vi "Serial.Get Com Port Device List.vi"(8 "error in":errorcluster) -> (0 "error out":errorcluster, 3 "Ports":T1(array[cluster]))   [LabVIEW 2018]
uses:
  <vilib>/KATE/Time/Time Utils.lvlib
panel:
  out "Duration(s)":dbl
  out "STD Error":string
  out "STD Out":string
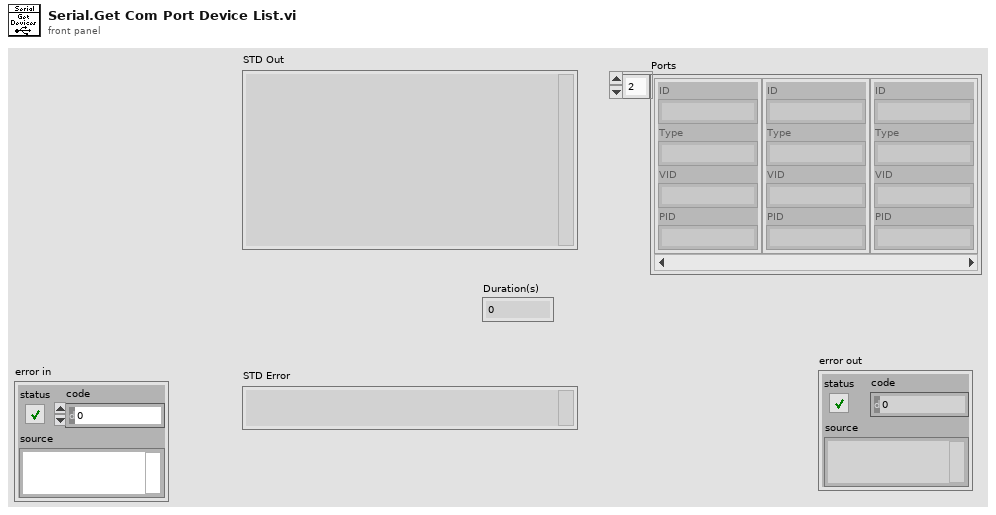
[diagram p1: front panel]
types:
  T1 = cluster{"ID":string, "Type":string, "VID":string, "PID":string}[]
  T2 = cluster{"ID":string, "Type":string, "VID":string, "PID":string}
  T3 = cluster{"STDIO":string, "Ports":cluster{"ID":string, "Type":string, "VID":string, "PID":string}[]}
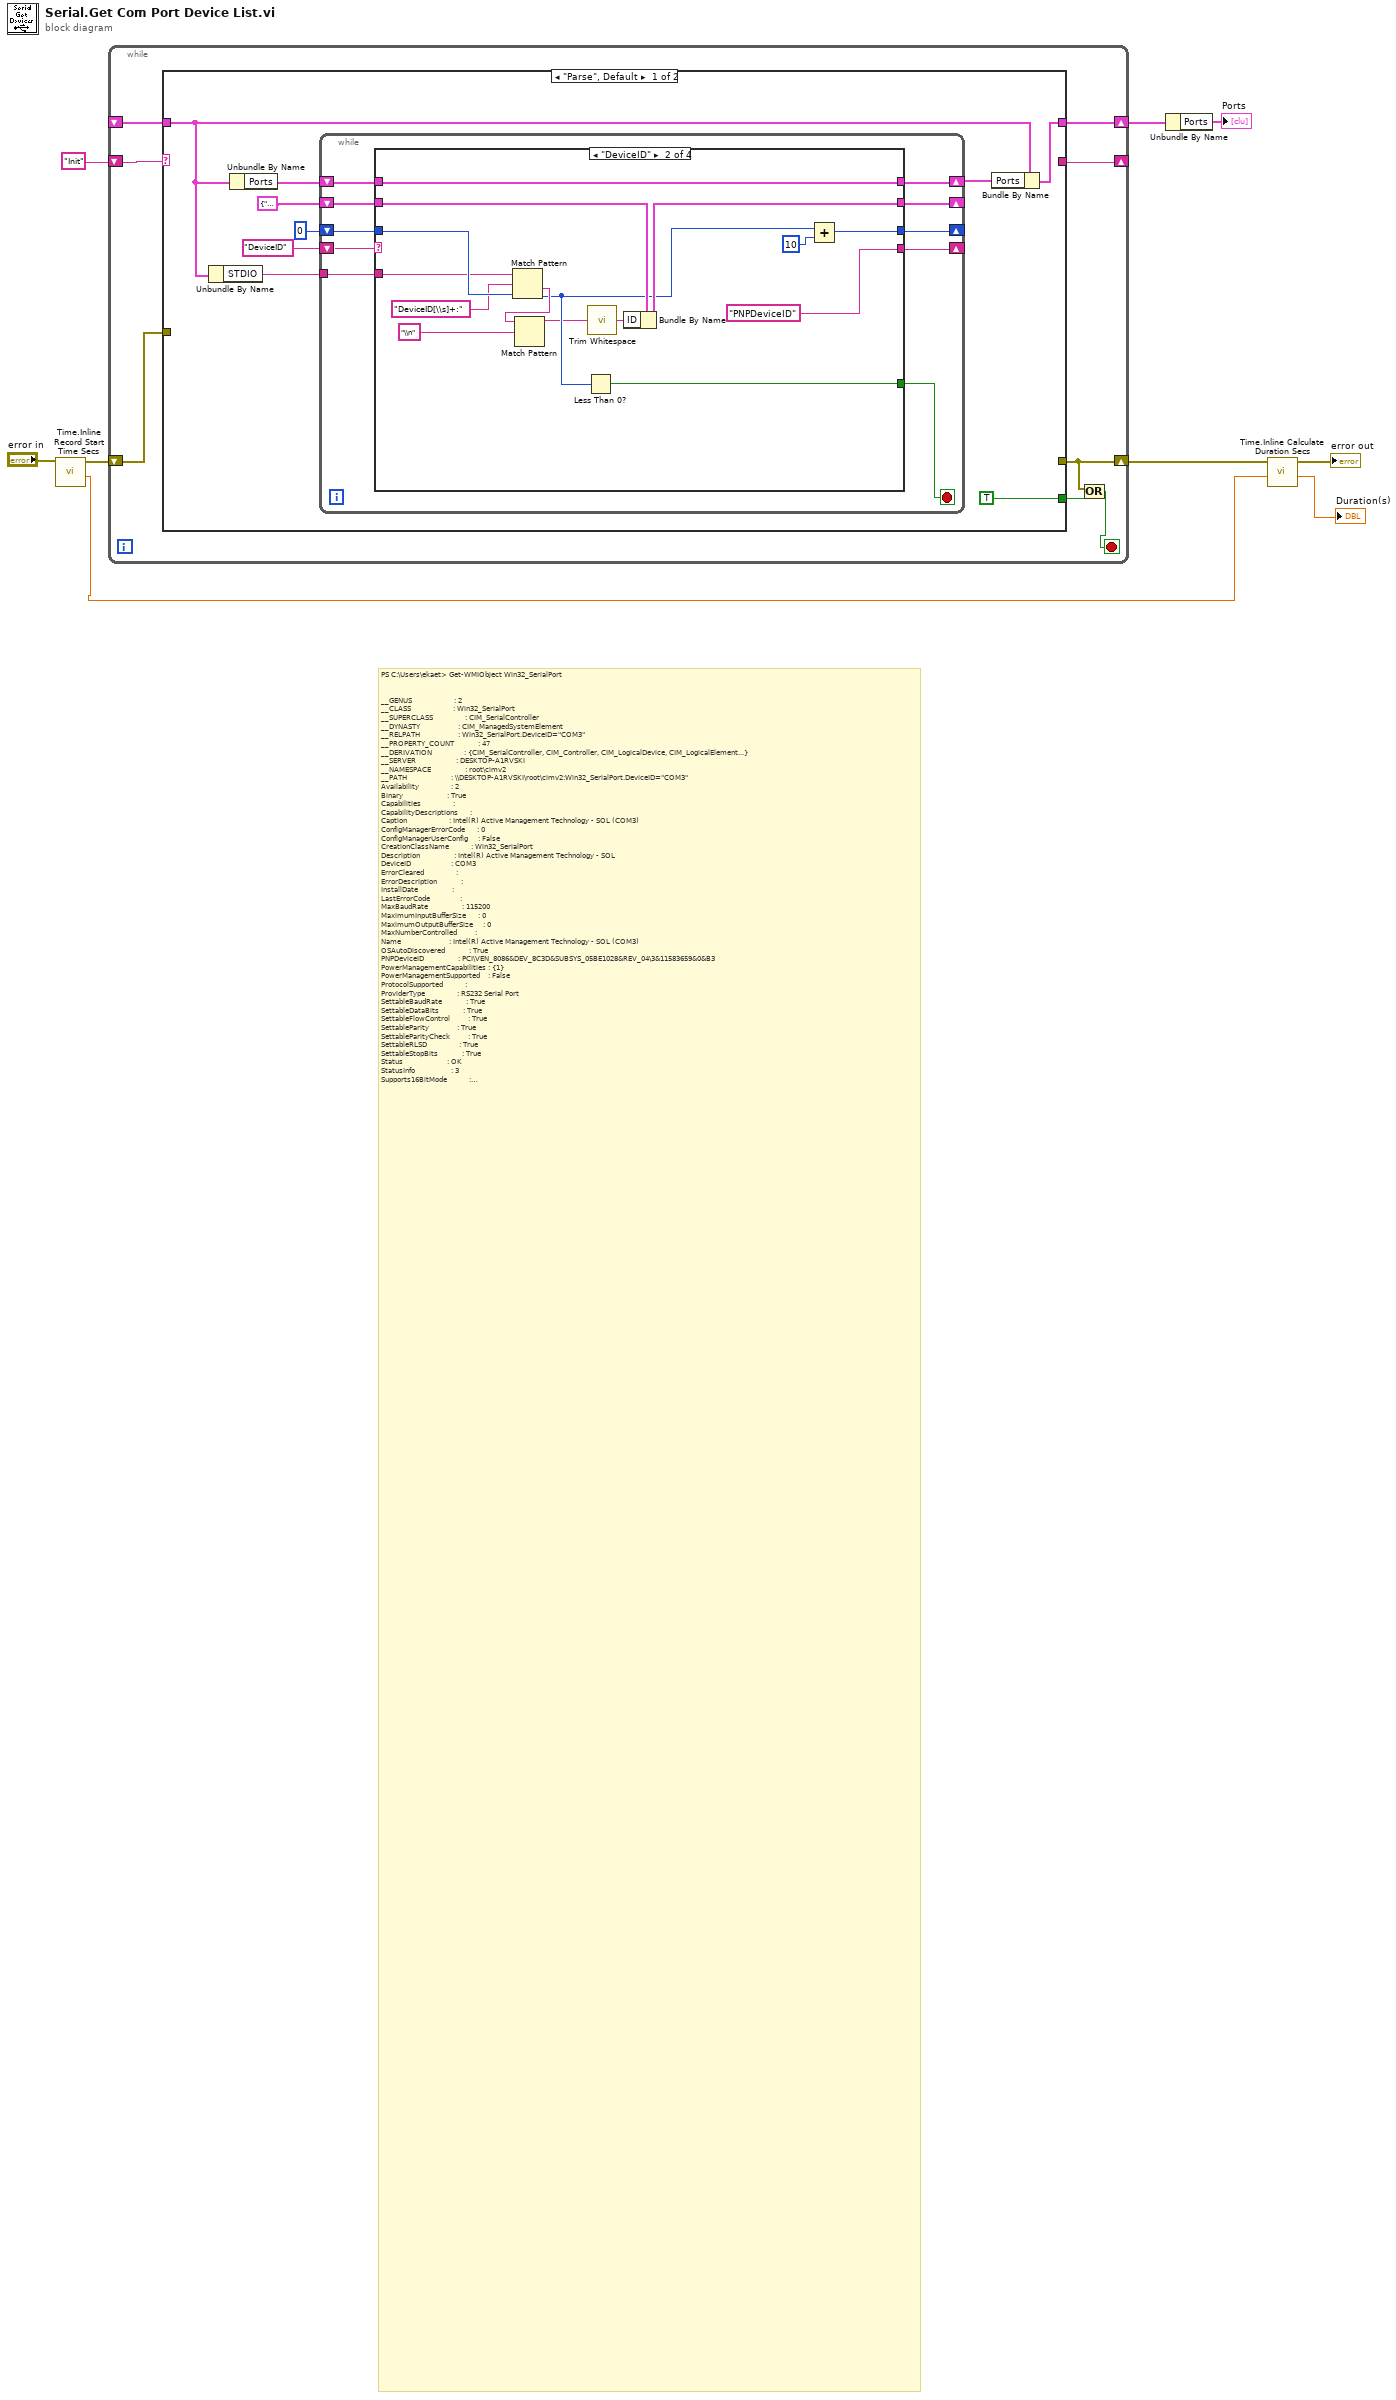
[diagram p0: block diagram]
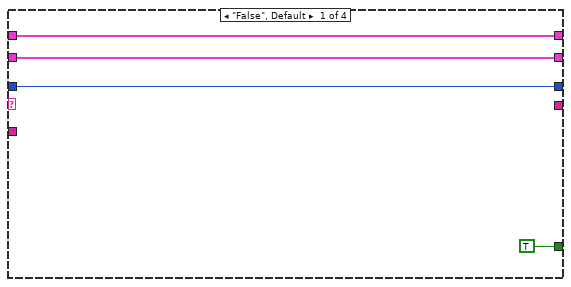
[diagram p2: hidden frame]
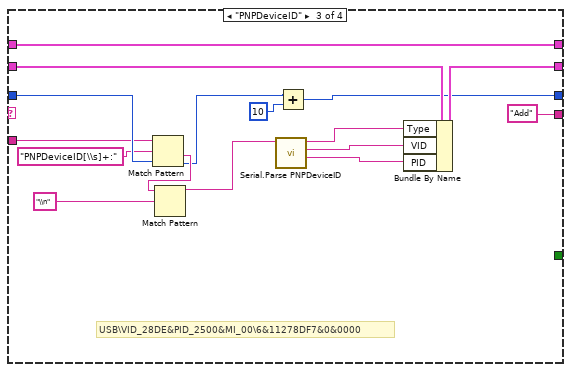
[diagram p3: hidden frame]
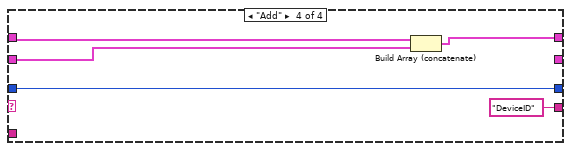
[diagram p4: hidden frame]
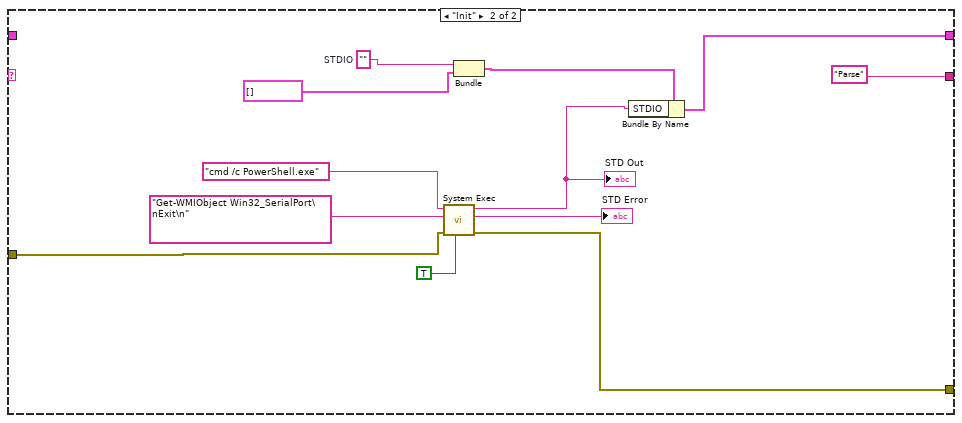
[diagram p5: hidden frame]
diagram:
  # "PS C:\\Users\\ekaet> Get-WMIObject Win32_SerialPort\n\n\n__GENUS                     : 2\n__CLASS                     : Win32_SerialPort\n__SUPERCLASS                : CIM_SerialController\n__DYNASTY                   : CIM_ManagedSystemElement\n__RELPATH                   : Win32_SerialPort.DeviceID=\"COM3\"\n__PROPERTY_COUNT            : 47\n__DERIVATION                : {CIM_SerialController, CIM_Controller, CIM_LogicalDevice, CIM_LogicalElement...}\n__SERVER                    : DESKTOP-A1RVSKI\n__NAMESPACE                 : root\\cimv2\n__PATH                      : \\\\DESKTOP-A1RVSKI\\root\\cimv2:Win32_SerialPort.DeviceID=\"COM3\"\nAvailability                : 2\nBinary                      : True\nCapabilities                :\nCapabilityDescriptions      :\nCaption                     : Intel(R) Active Management Technology - SOL (COM3)\nConfigManagerErrorCode      : 0\nConfigManagerUserConfig     : False\nCreationClassName           : Win32_SerialPort\nDescription                 : Intel(R) Active Management Technology - SOL\nDeviceID                    : COM3\nErrorCleared                :\nErrorDescription            :\nInstallDate                 :\nLastErrorCode               :\nMaxBaudRate                 : 115200\nMaximumInputBufferSize      : 0\nMaximumOutputBufferSize     : 0\nMaxNumberControlled         :\nName                        : Intel(R) Active Management Technology - SOL (COM3)\nOSAutoDiscovered            : True\nPNPDeviceID                 : PCI\\VEN_8086&DEV_8C3D&SUBSYS_05BE1028&REV_04\\3&11583659&0&B3\nPowerManagementCapabilities : {1}\nPowerManagementSupported    : False\nProtocolSupported           :\nProviderType                : RS232 Serial Port\nSettableBaudRate            : True\nSettableDataBits            : True\nSettableFlowControl         : True\nSettableParity              : True\nSettableParityCheck         : True\nSettableRLSD                : True\nSettableStopBits            : True\nStatus                      : OK\nStatusInfo                  : 3\nSupports16BitMode           : False\nSupportsDTRDSR              : True\nSupportsElapsedTimeouts     : True\nSupportsIntTimeouts         : True\nSupportsParityCheck         : True\nSupportsRLSD                : True\nSupportsRTSCTS              : True\nSupportsSpecialCharacters   : False\nSupportsXOnXOff             : True\nSupportsXOnXOffSet          : True\nSystemCreationClassName     : Win32_ComputerSystem\nSystemName                  : DESKTOP-A1RVSKI\nTimeOfLastReset             :\nPSComputerName              : DESKTOP-A1RVSKI\n\n__GENUS                     : 2\n__CLASS                     : Win32_SerialPort\n__SUPERCLASS                : CIM_SerialController\n__DYNASTY                   : CIM_ManagedSystemElement\n__RELPATH                   : Win32_SerialPort.DeviceID=\"COM6\"\n__PROPERTY_COUNT            : 47\n__DERIVATION                : {CIM_SerialController, CIM_Controller, CIM_LogicalDevice, CIM_LogicalElement...}\n__SERVER                    : DESKTOP-A1RVSKI\n__NAMESPACE                 : root\\cimv2\n__PATH                      : \\\\DESKTOP-A1RVSKI\\root\\cimv2:Win32_SerialPort.DeviceID=\"COM6\"\nAvailability                : 2\nBinary                      : True\nCapabilities                :\nCapabilityDescriptions      :\nCaption                     : USB Serial Device (COM6)\nConfigManagerErrorCode      : 0\nConfigManagerUserConfig     : False\nCreationClassName           : Win32_SerialPort\nDescription                 : USB Serial Device\nDeviceID                    : COM6\nErrorCleared                :\nErrorDescription            :\nInstallDate                 :\nLastErrorCode               :\nMaxBaudRate                 : 115200\nMaximumInputBufferSize      : 0\nMaximumOutputBufferSize     : 0\nMaxNumberControlled         :\nName                        : USB Serial Device (COM6)\nOSAutoDiscovered            : True\nPNPDeviceID                 : USB\\VID_28DE&PID_2500&MI_00\\6&11278DF7&0&0000\nPowerManagementCapabilities : {1}\nPowerManagementSupported    : False\nProtocolSupported           :\nProviderType                : Modem Device\nSettableBaudRate            : True\nSettableDataBits            : True\nSettableFlowControl         : True\nSettableParity              : True\nSettableParityCheck         : True\nSettableRLSD                : True\nSettableStopBits            : True\nStatus                      : OK\nStatusInfo                  : 3\nSupports16BitMode           : False\nSupportsDTRDSR              : True\nSupportsElapsedTimeouts     : True\nSupportsIntTimeouts         : True\nSupportsParityCheck         : True\nSupportsRLSD                : True\nSupportsRTSCTS              : False\nSupportsSpecialCharacters   : False\nSupportsXOnXOff             : False\nSupportsXOnXOffSet          : False\nSystemCreationClassName     : Win32_ComputerSystem\nSystemName                  : DESKTOP-A1RVSKI\nTimeOfLastReset             :\nPSComputerName              : DESKTOP-A1RVSKI"
  n1 = call <vilib>:"Time.Inline Record Start Time Secs.vi"("Error In Upper"="error in") -> ("Start(s)"=w2:dbl, "Error Out Upper"=w5:errorcluster)  [unwired: 8 in, 1 out]
  n2 = while {
    shift-right: [w14] -> w3
    shift-left: w5 -> [w17]
    shift-right: [w16] -> w8
    shift-left: _ -> [w12]
    shift-right: [w13] -> _
    shift-left: "Init" -> [w15]
    stop <- w10 stop-if-true
    n3 = case shown="\"Parse\", Default" w15 {
      tunnel: w17 -> [_ w85]
      tunnel: [_ w84] -> w14
      tunnel: [w19 w79] -> w16
      tunnel: [_ "Parse"] -> w13
      tunnel: w12 -> [w20 _]
      tunnel: [TRUE _] -> w11
      frame "Parse", Default {
        n4 = Unbundle By Name(w20) -> ("STDIO"=w25:string)
        n5 = Unbundle By Name(w20) -> ("Ports"=w22:T1)
        n6 = while {
          shift-right: [w34] -> w18
          shift-left: w22 -> [w35]
          shift-right: [w28] -> _
          shift-left: "DeviceID" -> [w36]
          shift-right: [w31] -> _
          shift-left: 0 -> [w32]
          tunnel: w25 -> [w33]
          shift-right: [w29] -> _
          shift-left: T2 {"ID"="", "Type"="", "VID"="", "PID"=""} ("Cluster") -> [w30]
          stop <- w27 stop-if-true
          n7 = case shown="\"DeviceID\"" w36 {
            tunnel: w35 -> [w39 w55 w71 w74]
            tunnel: [w39 w55 w71 w72] -> w34
            tunnel: w33 -> [_ w47 w60 _]
            tunnel: w32 -> [w40 w54 w70 w76]
            tunnel: [w40 w44 w57 w76] -> w31
            tunnel: w30 -> [w38 w51 w67 w73]
            tunnel: [w38 w50 w66 _] -> w29
            tunnel: [_ "PNPDeviceID" "Add" "DeviceID"] -> w28
            tunnel: [TRUE w48 _ _] -> w27
            frame "False", Default {
            }
            frame "DeviceID" {
              n8 = Match Pattern(string=w47, regular expression="DeviceID[\\s]+:", offset (0)=w54) -> (after substring=w46:string, offset past match=w43:i32)  [unwired: 2 out]
              n9 = Match Pattern(string=w46, regular expression="\\n") -> (before substring=w41:string)  [unwired: 1 in, 3 out]
              n10 = Less Than 0?(x=w43) -> (x < 0?=w48:bool)
              n11 = call <vilib>:"Trim Whitespace.vi"("string"=w41) -> ("trimmed string"=w42:string)  [unwired: 1 in]
              n12 = Bundle By Name(cluster=w51, "ID"=w42) -> (w50:T2)
              n13 = Add(x=w43, y=10) -> (x+y=w44:i32)
            }
            frame "PNPDeviceID" {
              # "USB\\VID_28DE&PID_2500&MI_00\\6&11278DF7&0&0000"
              n14 = Match Pattern(string=w60, regular expression="PNPDeviceID[\\s]+:", offset (0)=w70) -> (after substring=w59:string, offset past match=w58:i32)  [unwired: 2 out]
              n15 = Match Pattern(string=w59, regular expression="\\n") -> (before substring=w64:string)  [unwired: 1 in, 3 out]
              n16 = call "Serial.Parse PNPDeviceID.vi"("String"=w64) -> ("PID"=w61:string, "VID"=w62:string, "Type"=w63:string)  [unwired: 8 in]
              n17 = Add(x=w58, y=10) -> (x+y=w57:i32)
              n18 = Bundle By Name(cluster=w67, "Type"=w63, "VID"=w62, "PID"=w61) -> (w66:T2)
            }
            frame "Add" {
              n19 = Build Array (concatenate)(w74, w73) -> (w72:T1)
            }
          }
        }
        n20 = Bundle By Name(cluster=w20, "Ports"=w18) -> (w19:T3)
      }
      frame "Init" {
        w83 = ""  # STDIO
        n21 = call <vilib>:"System Exec.vi"("run minimized? (F)"=TRUE, "error in (no error)"=w85, "standard input"="Get-WMIObject Win32_SerialPort\nExit\n", "command line"="cmd /c PowerShell.exe") -> ("error out"=w84:errorcluster, "standard error"=→"STD Error":string, "standard output"=w80:string)  [unwired: 4 in, 1 out]
        "STD Out" <- w80
        n22 = Bundle("STDIO"=w83, "Ports"=T1 []) -> (w81:T3)  [unwired: 1 in]
        n23 = Bundle By Name(cluster=w81, "STDIO"=w80) -> (w79:T3)
      }
    }
    n24 = Or(x=w14, y=w11) -> (x .or. y?=w10:bool)
  }
  n25 = Unbundle By Name(w8) -> ("Ports"=→"Ports":T1)
  n26 = call <vilib>:"Time.Inline Calculate Duration Secs.vi"("Start(Sec)"=w2, "Error In Top"=w3) -> ("Duration(s)"=→"Duration(s)":dbl, "Error Out Top"=→"error out":errorcluster)  [unwired: 7 in, 1 out]
